vi "#5.vi"(0 "System no.":i32=1 min=1 max=4 step=1, 5 "error in":errorcluster) -> (14 "Axis moving?":bool[](array[boolean]), 19 "error out":errorcluster)   [LabVIEW 2026]
doc: "Polls the motion status of the connected axes by sending the single ASCII character 5. Connected axes are read from Global2.vi and displayed on the front panel for assignment. Required by General wait for movement to stop.vi and Wait for axes to stop.vi.\n\nAnalog: Motion status can only be determined for all connected axes, not for single axes.\n\nC-887, F-206: For GCS syntax version = GCS 1.0 (check with CSV?.vi. If CSV?.vi is not supported, syntax version is GCS 1.0) coding in answer is different, please use #5_old.vi.\n\nC-887, M-8X0: For GCS syntax version = GCS 1.0 (check with CSV?.vi. If CSV?.vi is not supported, syntax version is GCS 1.0) coding in answer is different, please use #5_old.vi."
panel:
  out "Connected axes":string[](array[string])
  # "Polls the motion status of the connected axes."
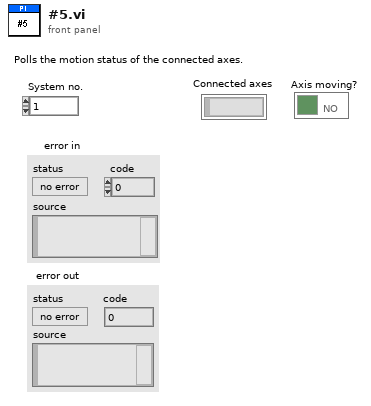
[diagram p1: front panel]
types:
  T1 = enum16{"Disable error check", "Force error check", "Use global settings"}
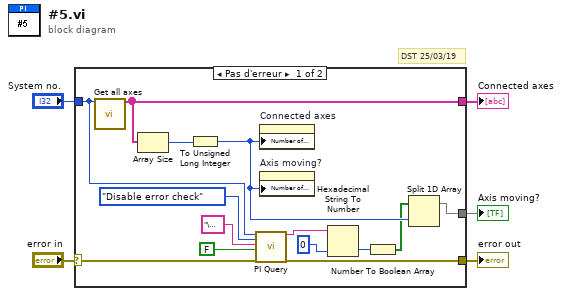
[diagram p0: block diagram]
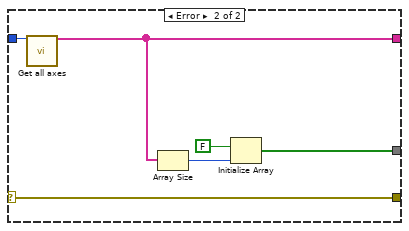
[diagram p2: hidden frame]
diagram:
  # "DST 25/03/19"
  n1 = case shown="Pas d'erreur" "error in" {
    selector: "error in" -> [w11 w25]
    tunnel: [w6 w21] -> w5
    tunnel: "System no." -> [w15 w24]
    tunnel: [w14 w23] -> w3
    tunnel: [w12 w25] -> w2
    frame No Error {
      n2 = call "Get all axes.vi"("System no."=w15) -> ("Conn. Axes"=w14:string[])  [unwired: 18 out]
      n3 = Array Size(array=w14) -> (size(s)=w17:i32)
      n4 = To Unsigned Long Integer(number=w17) -> (unsigned 32bit integer=w8:u32)
      n5 = call "PI Query.vi"("System no."=w15, "Error check settings"=T1."Disable error check", "String to send"="\u0005", "Attach termination char.?"=FALSE ("Attach Linefeed?"), "error in"=w11) -> ("String read"=w13:string, "error out"=w12:errorcluster)  [unwired: 2 in, 11 out]
      n6 = property on="Connected axes" class="Tabl (strict)"("Number of Rows"=w8) -> ()  [unwired: 2 in, 2 out]
      n7 = property on="Axis moving?" class="Tabl (strict)"("Number of Rows"=w8) -> ()  [unwired: 2 in, 2 out]
      n8 = Hexadecimal String To Number(string=w13, default (0uL)=u64 0) -> (number=w16:u64)  [unwired: 2 out]
      n9 = Number To Boolean Array(number=w16) -> (Boolean array=w7:bool[])
      n10 = Split 1D Array(array=w7, index=w8) -> (first subarray=w6:bool[])  [unwired: 1 out]
    }
    frame Error {
      n11 = call "Get all axes.vi"("System no."=w24) -> ("Conn. Axes"=w23:string[])  [unwired: 18 out]
      n12 = Array Size(array=w23) -> (size(s)=w22:i32)
      n13 = Initialize Array(FALSE, w22) -> (w21:bool[])
    }
  }
  "error out" <- w2
  "Axis moving?" <- w5
  "Connected axes" <- w3
